vi "Add_Image_Position_Offset.vi"() -> (5 "Plug in titles":string[](array[string]), 7 "Plug in values":string[](array[string]))   [LabVIEW 2015]
uses:
  Utilities/Image acquisition and processing/Feature detection/Typedefs/Theta range.ctl
  Utilities/Image acquisition and processing/Feature detection/Typedefs/Txy range.ctl
  Globals/Meas_global.vi
  Globals/Trav_pos_global.vi
  Globals/Extra_Commands_Global.vi
panel:
  out "Ty (pixels) Offset":dbl
  out "Tx (pixels) Offset":dbl
  out "Ty (pixels)":dbl
  out "Tx (pixels)":dbl
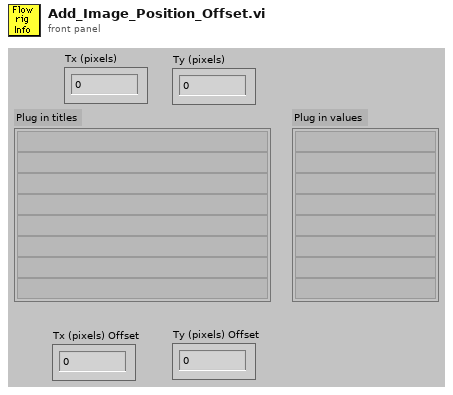
[diagram p1: front panel]
types:
  T1 = typedef "Theta range.ctl" = cluster{"theta max (deg)":dbl, "theta min (deg)":dbl}
  T2 = typedef "Txy range.ctl" = cluster{"Tx max (pix)":i32, "Tx min (pix)":i32, "Ty max (pix)":i32, "Ty min (pix)":i32}
  T3 = cluster{"Tx,y tol (abs pix)":dbl, "Rotation tol (abs deg)":dbl, "Scale tol (rel fact)":dbl}
  T4 = typedef "Traverse_cluster.ctl" = cluster{"Start X":sgl, "Start Y":sgl, "Start Z":sgl, "End X":sgl, "End Y":sgl, "End Z":sgl, "No. of pts.":i32, "Spacing":T5, "Filename":path, "Tunnel Speed":dbl, "Averaging time (min)":dbl, "Extra Commands":string, "Carrier_1 Q (l/min)":dbl, "Carrier_2 Q (l/min)":dbl, "Trace Gas Concentration (%)":dbl, "Specific Arguments":string, "Comments":string, "Row No":i32, "Row Type Selector":T6, "Completion time":string, "Row Duration (mins)":dbl, "No. of Valid pts.":i32, "Meas Setup File":string}
  T5 = typedef "Spacing.ctl" = enum16{"Linear", "Log", "Gauss", "Specified", "N/A"}
  T6 = typedef "Multi_run_mode.ctl" = enum16{"Move Traverse Only", "Set Tunnel Speed Only", "Set Source Only", "Set Measurement Conditions", "Single Measurement", "Vertical Profile", "Lateral Profile", "Longitudinal Profile", "Explore Volume", "Multi-Axis Profile", "Auto Calibrate", "Meas Fast FID Bkgnd", "Check Beam Power", "Scanning Valve Measurement", "Run VI Named:", "Set ADAM Ch", "Wait (minutes)", "Send Message", "Synchronize With:", "Fall Back to this Row", "Turn Off Row Repeating", "Blank Row", "Traverse 3D Volume"}
  T7 = typedef "ROI bounds.ctl" = cluster{"Xmax":i32, "Ymax":i32, "Xmin":i32, "Ymin":i32}
  T8 = typedef "Top level controls.ctl" = cluster{"Auto ROI (for rot.)":bool, "Apply scaling":bool, "Apply rotation":bool, "Apply Tx":bool, "Apply Ty":bool, "Keep proc. img":bool}
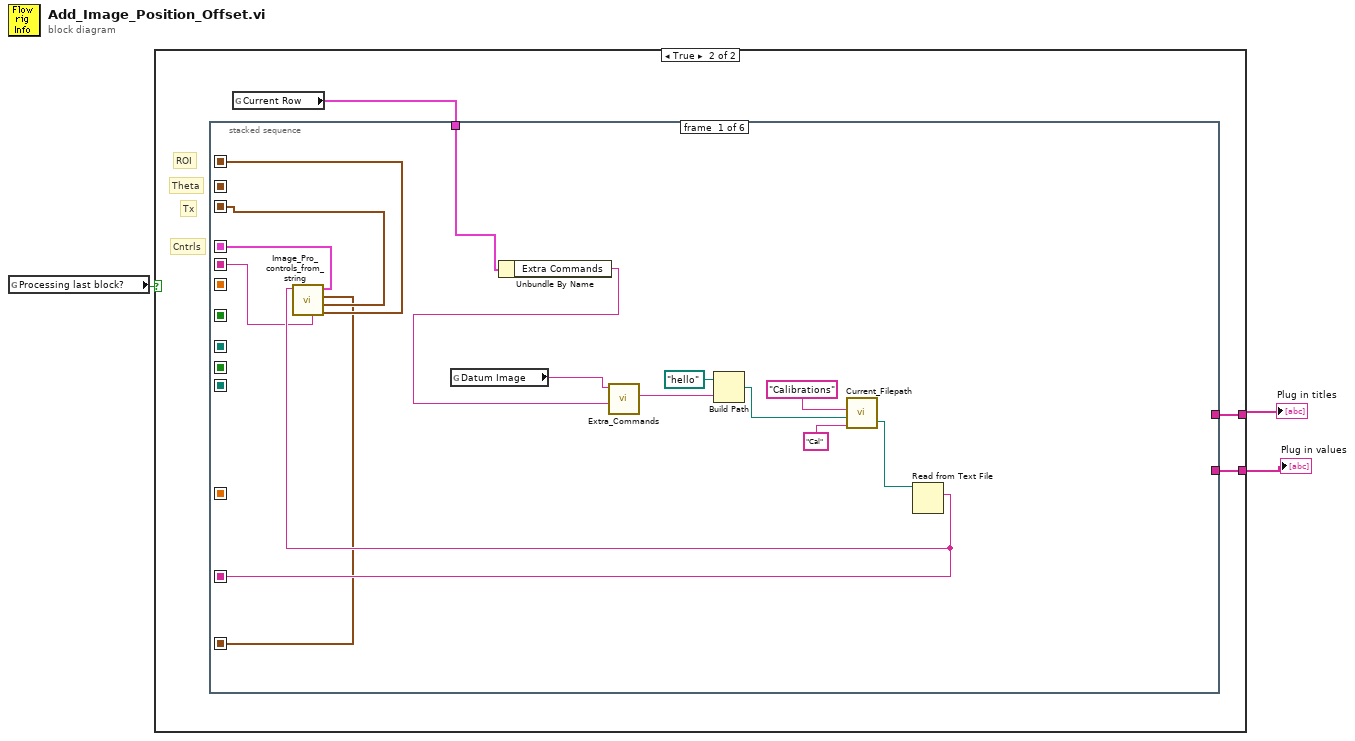
[diagram p0: block diagram]
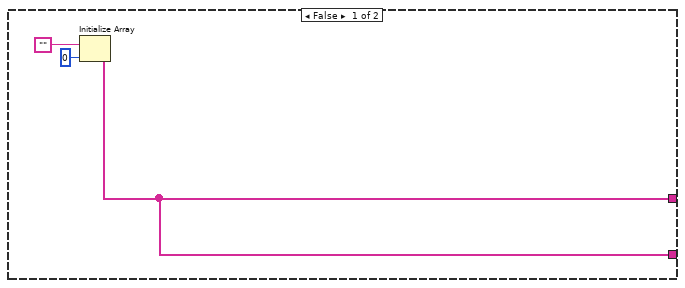
[diagram p2: hidden frame]
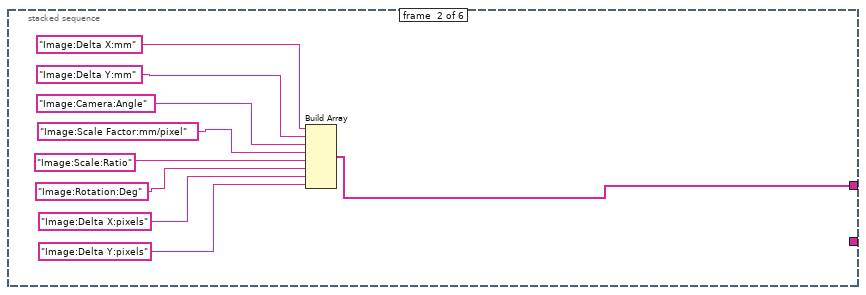
[diagram p3: hidden frame]
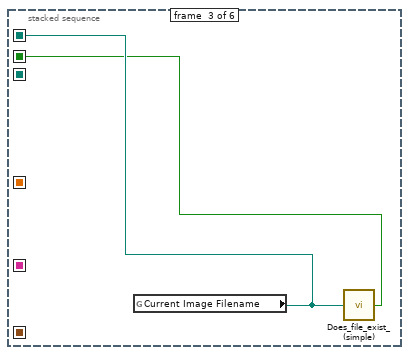
[diagram p4: hidden frame]
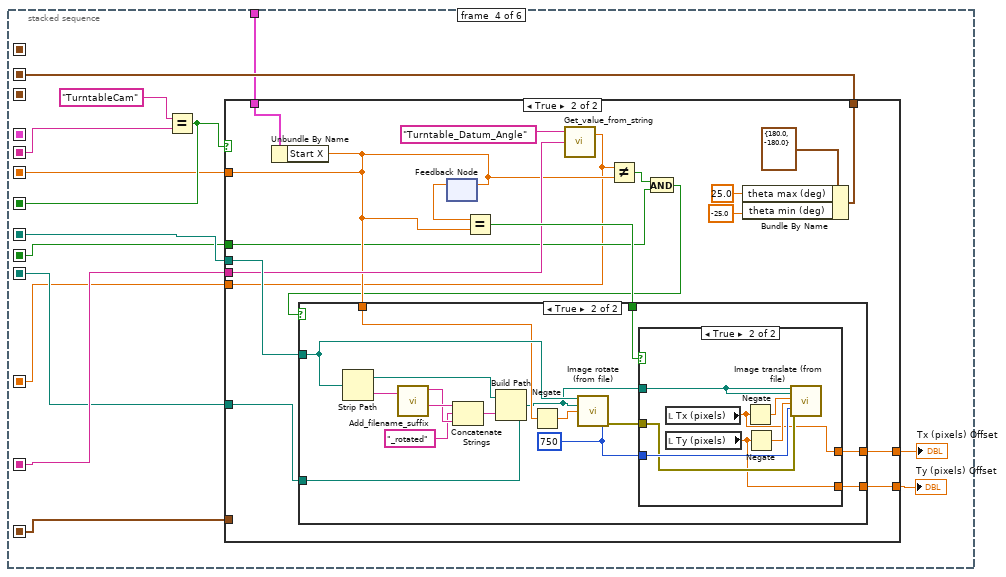
[diagram p5: hidden frame]
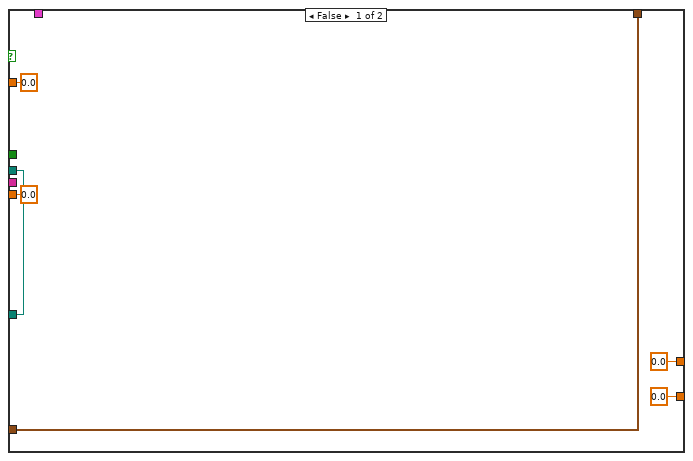
[diagram p6: hidden frame]
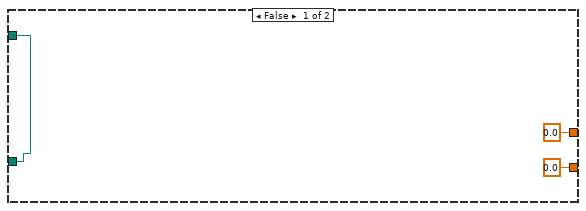
[diagram p7: hidden frame]
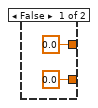
[diagram p8: hidden frame]
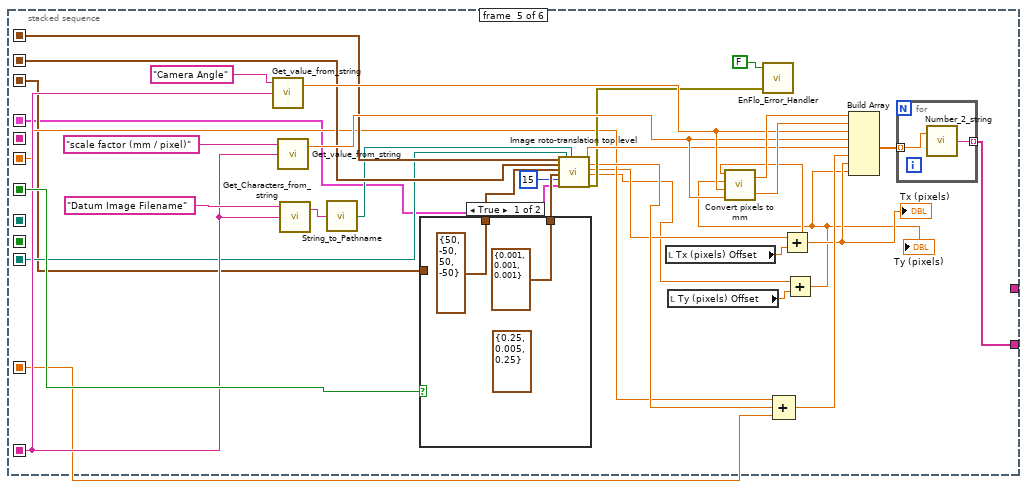
[diagram p9: hidden frame]
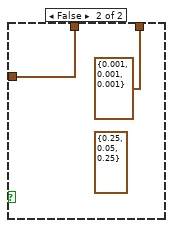
[diagram p10: hidden frame]
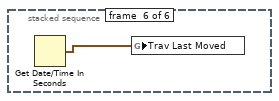
[diagram p11: hidden frame]
diagram:
  n1 = global read "Meas_global.vi" "Processing last block?"() -> (w3:bool)
  n2 = case shown="True" w3 {
    tunnel: [w4 w8] -> w2
    tunnel: [w4 w9] -> w1
    frame False {
      n3 = Initialize Array("", 0) -> (w4:string[])
    }
    frame True {
      # "Theta"
      # "Cntrls"
      # "Tx"
      # "ROI"
      n4 = global read "Trav_pos_global.vi" "Current Row"() -> (w7:T4)
      n5 = stacked-sequence {
        seq-local: [w15 _ _ _ _ _] -> [_ _ _ w48 w117 _]
        seq-local: [w12 _ _ _ _ _] -> [_ _ _ _ w124 _]
        seq-local: [_ _ _ w49 _ _] -> [_ _ _ _ w123 _]
        seq-local: [_ _ _ w46 _ _] -> [_ _ _ _ w118 _]
        seq-local: [_ _ _ w44 _ _] -> [_ _ _ _ w112 _]
        seq-local: [_ _ _ w43 _ _] -> [_ _ _ _ w113 _]
        seq-local: [w13 _ _ _ _ _] -> [_ _ _ _ w103 _]
        seq-local: [w14 _ _ _ _ _] -> [_ _ _ _ w102 _]
        seq-local: [_ _ w35 _ _ _] -> [_ _ _ w40 _ _]
        seq-local: [_ _ w34 _ _ _] -> [_ _ _ w39 _ _]
        seq-local: [_ _ _ w38 _ _] -> [_ _ _ _ w101 _]
        seq-local: [w11 _ _ _ _ _] -> [_ _ _ w36 _ _]
        seq-local: [w10 _ _ _ _ _] -> [_ _ _ w37 _ _]
        tunnel: [_ _ _ _ w125 _] -> w9
        tunnel: [_ w25 _ _ _ _] -> w8
        tunnel: w7 -> [w16 _ _ w45 _ _]
        frame #0 {
          n6 = global read "Extra_Commands_Global.vi" "Datum Image"() -> (w24:string)
          n7 = Unbundle By Name(w16) -> ("Extra Commands"=w23:string)
          n8 = call "Extra_Commands.vi"("String to Search"=w23, "Command"=w24) -> ("String Value"=w18:string)  [unwired: 1 in, 4 out]
          n9 = Build Path(base path=path "hello", name or relative path=w18) -> (appended path=w22:path)
          n10 = call "Current_Filepath.vi"("Short_Name"="Cal" ("Data Type"), "Filename in"=w22, "Data Type"="Calibrations") -> ("Filename Out"=w17:path)  [unwired: 1 in, 1 out]
          n11 = Read from Text File(file (use dialog)=w17) -> (text=w15:string)  [unwired: 3 in, 3 out]
          n12 = call "Image_Pro_controls_from_string.vi"("Setup String"=w15) -> ("ROI to crop (pixels)"=w12:T7, "Txy range (pixels)"=w13:T2, "Theta range (deg)"=w10:T1, "Controls"=w14:T8, "Camera"=w11:string)  [unwired: 6 in]
        }
        frame #1 {
          n13 = Build Array("Image:Delta X:mm", "Image:Delta Y:mm", "Image:Camera:Angle", "Image:Scale Factor:mm/pixel", "Image:Scale:Ratio", "Image:Rotation:Deg", "Image:Delta X:pixels", "Image:Delta Y:pixels") -> (w25:string[])
        }
        frame #2 {
          n14 = global read "Trav_pos_global.vi" "Current Image Filename"() -> (w35:path)
          n15 = call "Does_file_exist_(simple).vi"("Pathname"=w35) -> ("exists?"=w34:bool)
        }
        frame #3 {
          n16 = Equal?(x="TurntableCam", y=w36) -> (x = y?=w46:bool)
          n17 = case shown="True" w46 {
            tunnel: [w50 w72] -> w49
            tunnel: w48 -> [_ w61]
            tunnel: w45 -> [_ w69]
            tunnel: [w55 w68] -> w44
            tunnel: w40 -> [w55 w67]
            tunnel: [sgl 0.0 ("Start X") w60] -> w43
            tunnel: [0.0 ("Ty (pixels)") w64] -> w42
            tunnel: [0.0 ("Tx (pixels)") w63] -> w41
            tunnel: w39 -> [_ w58]
            tunnel: [0.0 ("Value") w56] -> w38
            tunnel: w37 -> [w50 _]
            frame False {
            }
            frame True {
              n18 = Unbundle By Name(w69) -> ("Start X"=w60:sgl)
              n19 = feedback-in #1(w60) -> ()
              n20 = feedback #1() -> (w66:sgl)  [unwired: 1 in]
              n21 = Equal?(x=w66, y=w60) -> (x = y?=w65:bool)
              n22 = call "Get_value_from_string.vi"("Input string"=w61, "Variable name"="Turntable_Datum_Angle" ("Label for value")) -> ("Value"=w56:dbl)  [unwired: 1 in, 1 out]
              n23 = Not Equal?(x=w56, y=w60) -> (x != y?=w59:bool)
              n24 = And(x=w59, y=w58) -> (x .and. y?=w57:bool)
              n25 = case shown="True" w57 {
                tunnel: [w76 w82] -> w68
                tunnel: w67 -> [w76 w85]
                tunnel: w60 -> [_ w83]
                tunnel: w65 -> [_ w79]
                tunnel: [0.0 ("Ty (pixels)") w78] -> w64
                tunnel: [0.0 ("Tx (pixels)") w77] -> w63
                frame False {
                }
                frame True {
                  w81 = u32 750 ("Quality")
                  n26 = Strip Path(path=w85) -> (stripped path=w86:path, name=w91:string)
                  n27 = call "Add_filename_suffix.vi"("Filename"=w91) -> ("Original Suffix"=w89:string, "Base name"=w90:string)  [unwired: 1 in, 2 out]
                  n28 = Concatenate Strings(w90, "_rotated" ("string"), w89) -> (w87:string)
                  n29 = Build Path(base path=w86, name or relative path=w87) -> (appended path=w82:path)
                  n30 = Negate(x=w83) -> (-x=w84:sgl)
                  n31 = call "Image rotate (from file).vi"("Image file path"=w85, "Rotated image file path"=w82, "Rotation angle, ccw+ (deg)"=w84, "Quality"=w81) -> ("Error Out"=w80:errorcluster)  [unwired: 11 in]
                  n32 = case shown="True" w79 {
                    tunnel: w82 -> [_ w98]
                    tunnel: w81 -> [_ w100]
                    tunnel: w80 -> [_ w99]
                    tunnel: [0.0 ("Ty (pixels)") w95] -> w78
                    tunnel: [0.0 ("Tx (pixels)") w94] -> w77
                    frame False {
                    }
                    frame True {
                      n33 = local read "Tx (pixels)"() -> (w94:dbl)
                      n34 = local read "Ty (pixels)"() -> (w95:dbl)
                      n35 = Negate(x=w94) -> (-x=w97:dbl)
                      n36 = Negate(x=w95) -> (-x=w96:dbl)
                      n37 = call "Image translate (from file).vi"("Image file path"=w98, "Translated image file path"=w98, "Tx (pixels)"=w97, "Ty (pixels)"=w96, "Quality"=w100, "Error in"=w99) -> ()  [unwired: 13 in, 1 out]
                    }
                  }
                }
              }
              n38 = Bundle By Name(cluster=T1 {"theta max (deg)"=180.0, "theta min (deg)"=-180.0} ("Theta range (deg)"), "theta max (deg)"=25.0, "theta min (deg)"=-25.0) -> (w72:T1)
            }
          }
          "Tx (pixels) Offset" <- w41
          "Ty (pixels) Offset" <- w42
        }
        frame #4 {
          n39 = call "Get_value_from_string.vi"("Input string"=w117, "Variable name"="Camera Angle" ("Label for value")) -> ("Value"=w128:dbl)  [unwired: 1 in, 1 out]
          n40 = call "Get_value_from_string.vi"("Input string"=w117, "Variable name"="scale factor (mm / pixel)" ("Label for value")) -> ("Value"=w127:dbl)  [unwired: 1 in, 1 out]
          n41 = call "Get_Characters_from_string.vi"("Input string"=w117, "Variable name"="Datum Image Filename" ("Label for characters")) -> ("Value"=w131:string)  [unwired: 1 in, 1 out]
          n42 = call "String_to_Pathname.vi"("Input String"=w131) -> ("path"=w121:path)
          n43 = case shown="True" w118 {
            tunnel: [T3 {"Tx,y tol (abs pix)"=0.001, "Rotation tol (abs deg)"=0.001, "Scale tol (rel fact)"=0.001} ("Convergence tolerances") T3 {"Tx,y tol (abs pix)"=0.001, "Rotation tol (abs deg)"=0.001, "Scale tol (rel fact)"=0.001} ("Convergence tolerances")] -> w114
            tunnel: [T2 {"Tx max (pix)"=50, "Tx min (pix)"=-50, "Ty max (pix)"=50, "Ty min (pix)"=-50} ("Txy range (pixels)") w137] -> w111
            tunnel: w103 -> [_ w137]
            frame True {
              (unwired) T3 {"Tx,y tol (abs pix)"=0.25, "Rotation tol (abs deg)"=0.005, "Scale tol (rel fact)"=0.25} ("Convergence tolerances")
            }
            frame False {
              (unwired) T3 {"Tx,y tol (abs pix)"=0.25, "Rotation tol (abs deg)"=0.05, "Scale tol (rel fact)"=0.25} ("Convergence tolerances")
            }
          }
          n44 = call "Image roto-translation top level.vi"("ROI to crop (pixels)"=w124, "Theta range (deg)"=w123, "Txy range (pixels)"=w111, "Convergence tolerances"=w114, "Max. iters"=15, "Controls"=w102, "Test image file path"=w112, "Reference image file path"=w121) -> ("Scale factor"=w122:dbl, "Rotation (deg)"=w116:dbl, "Tx (pixels)"=w109:dbl, "Ty (pixels)"=w106:dbl, "Error Out"=w120:errorcluster)  [unwired: 5 in, 2 out]
          n45 = local read "Tx (pixels) Offset"() -> (w110:dbl)
          n46 = local read "Ty (pixels) Offset"() -> (w108:dbl)
          n47 = call "EnFlo_Error_Handler.vi"("error in (no error)"=w120, "Dialog Box (T)"=FALSE) -> ()  [unwired: 1 in, 3 out]
          n48 = Compound Arithmetic op=ADD(w113, w116, w101) -> (w115:dbl)
          n49 = Add(x=w109, y=w110) -> (x+y=w107:dbl)
          "Tx (pixels)" <- w107
          n50 = Add(x=w106, y=w108) -> (x+y=w105:dbl)
          "Ty (pixels)" <- w105
          n51 = call "Convert pixels to mm.vi"("scale factor (mm / pixel)"=w127, "camera angle, ccw+ rel. to trav. (deg)"=w128, "dy (pix)"=w105, "dx (pix)"=w107) -> ("dy (mm)"=w129:dbl, "dx (mm)"=w130:dbl)
          n52 = Build Array(w130, w129, w128, w127, w122, w115, w107, w105) -> (w126:dbl[])
          n53 = for {
            tunnel: w126 -> [w140] mode=indexing
            tunnel: [w139] -> w125 mode=indexing
            n54 = call "Number_2_string.vi"("number"=w140) -> ("String"=w139:string)  [unwired: 1 in]
          }
        }
        frame #5 {
          n55 = Get Date/Time In Seconds() -> (seconds since 1Jan1904=w141:timestamp)
          n56 = global write "Trav_pos_global.vi" "Trav Last Moved"(w141) -> ()
        }
      }
    }
  }
  "Plug in titles" <- w2
  "Plug in values" <- w1
